vi "Read.vi"(7 "timeout (100ms)":i32=100, 8 "error in (no error)":errorcluster, 9 "Interlock in":bool, 11 "Interlock I32 in":refnum<class "IL I32 Pass.lvclass">) -> (0 "error out":errorcluster, 1 "Interlock out":bool, 2 "Data out":variant, 3 "Interlock I32 out":refnum<class "IL I32 Pass.lvclass">, 4 "IL Action":refnum<class "IL Action.lvclass">[](array[class]))   [LabVIEW 2015, in "Interlocks.lvlib" / "IL I32 Pass.lvclass"]
uses:
  IL I32 Pass.lvclass
  IL Action/IL Action.lvclass
  IL I32 Pass.lvclass/IL I32 Pass.ctl
  Interlock/State Enum.ctl
  Interlock/Interlock.lvclass/Interlock.ctl
  Interlock/Interlock.lvclass
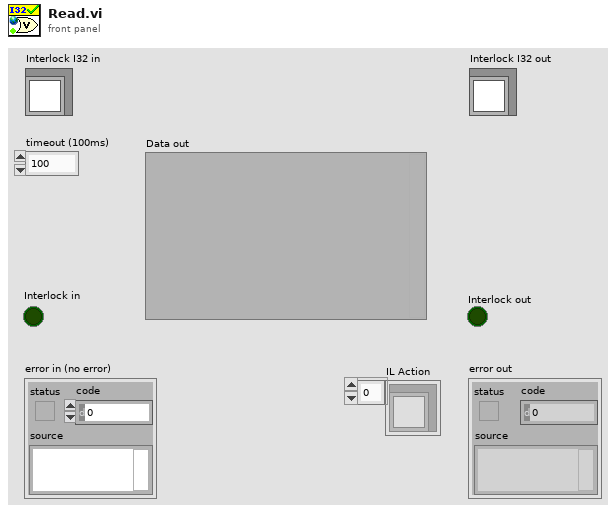
[diagram p1: front panel]
types:
  T1 = typedef "Interlocks.lvlib/Interlock.lvclass/State Enum.ctl" = enum16{"Error", "Ok", "Interlock", "Out of Range", "Is ON", "Is OFF", "Denied", "Not Allowed", "Sample Allow", "Sample Deny"}
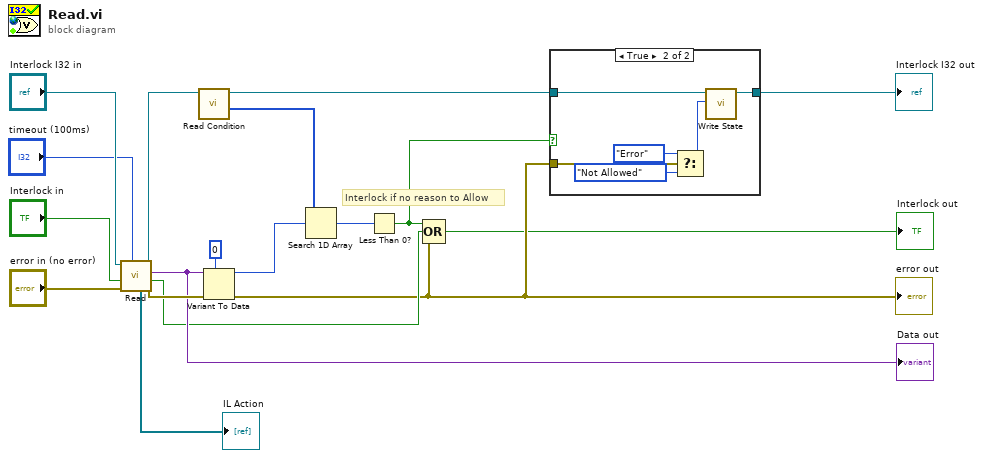
[diagram p0: block diagram]
diagram:
  # "Interlock if no reason to Allow"
  n1 = call-parent "Read.vi"("timeout (100ms)"="timeout (100ms)", "error in (no error)"="error in (no error)", 9:"Interlock in"="Interlock in", 11:"Interlock in"="Interlock I32 in") -> ("error out"=w15:errorcluster, 1:"Interlock out"=w8:bool, "Data out"=w12:variant, 3:"Interlock out"=w13:refnum<class "IL I32 Pass.lvclass">, "IL Action"=→"IL Action":refnum<class "IL Action.lvclass">[])  [unwired: 3 in]
  "Data out" <- w12
  n2 = call "Read Condition.vi"("Interlock I32 in"=w13) -> ("Allow"=w11:i32[], "Interlock I32 out"=w4:refnum<class "IL I32 Pass.lvclass">)  [unwired: 9 in]
  n3 = Variant To Data(error in=w15, type=0, Variant=w12) -> (data=w10:i32, error out=w7:errorcluster)
  "error out" <- w7
  n4 = Search 1D Array(1D array=w11, element=w10) -> (index of element=w9:i32)  [unwired: 1 in]
  n5 = Less Than 0?(x=w9) -> (x < 0?=w5:bool)
  n6 = Compound Arithmetic op=OR(w5, w8, w7) -> (→"Interlock out":bool)
  n7 = case shown="True" w5 {
    tunnel: w7 -> [_ w25]
    tunnel: w4 -> [w19 w22]
    tunnel: [w19 w21] -> w3
    frame False {
    }
    frame True {
      n8 = Select(t=State_Enum."Error", s=w25, f=State_Enum."Not Allowed" ("State")) -> (s? t:f=w20:T1)
      n9 = call "Write State.vi"("State"=w20, "Interlock in"=w22) -> ("Interlock out"=w21:refnum<class "IL I32 Pass.lvclass">)  [unwired: 9 in]
    }
  }
  "Interlock I32 out" <- w3
